vi "禁用控件.vi"(7 "禁用？(F)":bool, 8 "错误输入（无错误）":errorcluster, 11 "本VI":refnum<vi>) -> (0 "错误输出":errorcluster)   [LabVIEW 2020]
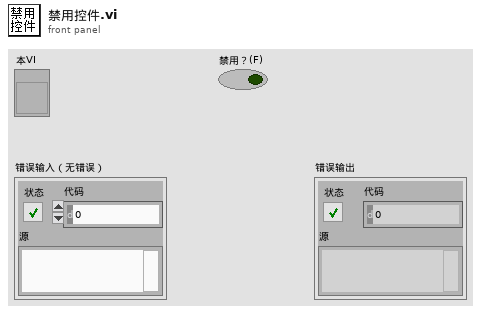
[diagram p1: front panel]
types:
  T1 = enum8{"Enabled", "Disabled", "Disabled and Grayed Out"}
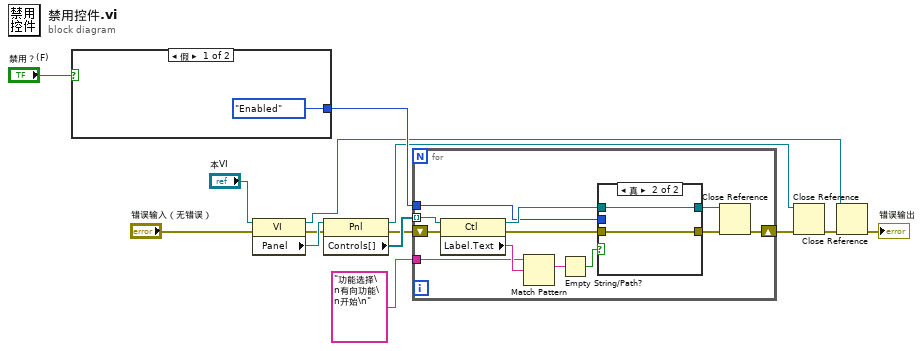
[diagram p0: block diagram]
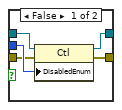
[diagram p2: hidden frame]
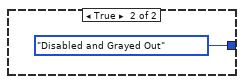
[diagram p3: hidden frame]
diagram:
  n1 = case shown="假" "禁用？(F)" {
    tunnel: [T1."Enabled" ("禁用") T1."Disabled and Grayed Out" ("禁用")] -> w10
    frame False {
    }
    frame True {
    }
  }
  n2 = property class="VI"(reference="本VI", error in="错误输入（无错误）") -> (reference out=w7:refnum<vi>, error out=w5:errorcluster, "Panel"=w13:refnum<vi>)
  n3 = property class="Pnl"(reference=w13, error in=w5) -> (reference out=w8:refnum<vi>, error out=w4:errorcluster, "Controls[]"=w12:refnum<vi>[])
  n4 = for {
    tunnel: w12 -> [w28] mode=indexing
    tunnel: "功能选择\n有向功能\n开始\n" -> [w26]
    tunnel: w10 -> [w22]
    shift-right: [w17] -> w3
    shift-left: w4 -> [w20]
    n5 = property class="Ctl"(reference=w28, error in=w20) -> (reference out=w23:refnum<vi>, error out=w19:errorcluster, "Label.Text"=w27:string)
    n6 = Match Pattern(string=w26, regular expression=w27) -> (match substring=w25:string)  [unwired: 1 in, 3 out]
    n7 = Empty String/Path?(string/path=w25) -> (empty?=w24:bool)
    n8 = case shown="真" w24 {
      tunnel: w23 -> [w33 w35]
      tunnel: w22 -> [w32 _]
      tunnel: [w31 w35] -> w21
      tunnel: w19 -> [w30 w34]
      tunnel: [w29 w34] -> w18
      frame False {
        n9 = property class="Ctl"(reference=w33, error in=w30, "DisabledEnum"=w32) -> (reference out=w31:refnum<vi>, error out=w29:errorcluster)
      }
      frame True {
      }
    }
    n10 = Close Reference(reference=w21, error in (no error)=w18) -> (error out=w17:errorcluster)
  }
  n11 = Close Reference(reference=w8, error in (no error)=w3) -> (error out=w2:errorcluster)
  n12 = Close Reference(reference=w7, error in (no error)=w2) -> (error out=→"错误输出":errorcluster)
